vi "Main.vi"(11 "Module Admin":refnum<class "Delacor_lib_QMH_Module Admin.lvclass">) -> ()   [LabVIEW 2020, in "UI User.lvlib"]
doc: "This template is based off of the Queued Message Handler design pattern and the Queued Message Handler project template that ships with LabVIEW.\n\nThe main difference is that the queue is private to this module and communication between modules is performed via Broadcast and Request events.\n\nRequest events are wrapped in public API methods and are handled in the Event Handling Loop (EHL) of this VI. Any module can register for Broadcast events sent by this module. The EHL generates messages based on user interface actions.\n\nThe Message Handling Loop (MHL) processes messages generated by the EHL, or by other messages. The messages are string values, so new messages can be added easily to the Message Cases case structure in the MHL. Each message cluster can also provide an optional value for Message Data, which is a variant that can be converted to whatever message-specific data is required.\n_____\nBased on DQMH Project Template 6.0.0.91."
uses:
  UI User.lvlib
  <vilib>/Delacor/Delacor QMH/Libraries/Module Admin_class/Delacor_lib_QMH_Module Admin.lvclass
  Module Data--cluster.ctl
  Stop Argument--cluster.ctl
  <vilib>/Delacor/Delacor QMH/Libraries/Message Queue_class/Delacor_lib_QMH_Message Queue.lvclass/Delacor_lib_QMH_Message Queue.ctl
  <vilib>/Delacor/Delacor QMH/Libraries/Module Admin_class/Delacor_lib_QMH_Module Admin.lvclass/Delacor_lib_QMH_Module Admin.ctl
  <vilib>/Delacor/Delacor QMH/Libraries/Message Queue_class/Delacor_lib_QMH_Enqueue Message (Single).vi
  <vilib>/Delacor/Delacor QMH/Libraries/Module Admin_class/Delacor_lib_QMH_Get External Launch.vi
  <vilib>/Utility/error.llb/Error Cluster From Error Code.vi
  <vilib>/ErrorRing/Error Ring.xnode
  <vilib>/Delacor/Delacor QMH/Libraries/Message Queue_class/Delacor_lib_QMH_Message Queue.lvclass
  Hardware DAQ/Hardware DAQ.lvlib
  Client HTTP Post/Client HTTP Post.lvlib
  Client HTTP Get/Client HTTP Get.lvlib
panel:
  in  "Radio Buttons Main":T1(radio)
  out "Tab Main":T2(tab)
  out "Active Modules (GET)":string[](array[string])
  in  "ID GET":i32(ring) items=["All"=-1, "1"=1, "2"=2, "3"=3, "4"=4]
  in  "Arrancar - GET":bool
  out "Active Modules (POST)":string[](array[string])
  in  "ID POST":i32(ring) items=["All"=-1, "1"=1, "2"=2, "3"=3]
  in  "Arrancar - POST":bool
  in  "Open Panel DAQ":bool
  in  "Show Panel DAQ":bool
  out "Contador Productos":u16(knob) caption="Gauge" scale=0.0..250.0
  out "DO-3":bool
  out "DO-2":bool
  out "DO-1":bool
  out "DO-0":bool
  in  "Digital Output 3":bool
  in  "Digital Output 2":bool
  in  "Digital Output 1":bool
  in  "Digital Output 0":bool
  out "Digital Inputs":bool[](array[boolean])
  out "Voltimetro - 4":dbl format="%.3f"
  out "Voltimetro - 3":dbl format="%.3f"
  out "Voltimetro - 2":dbl format="%.3f"
  out "Voltimetro - 1":dbl format="%.3f"
  out "Radio Indicador":T3(radio)
  # "Sistema Para Pruebas de Medida (Hardware Embebido,\nHardware Industrial)"
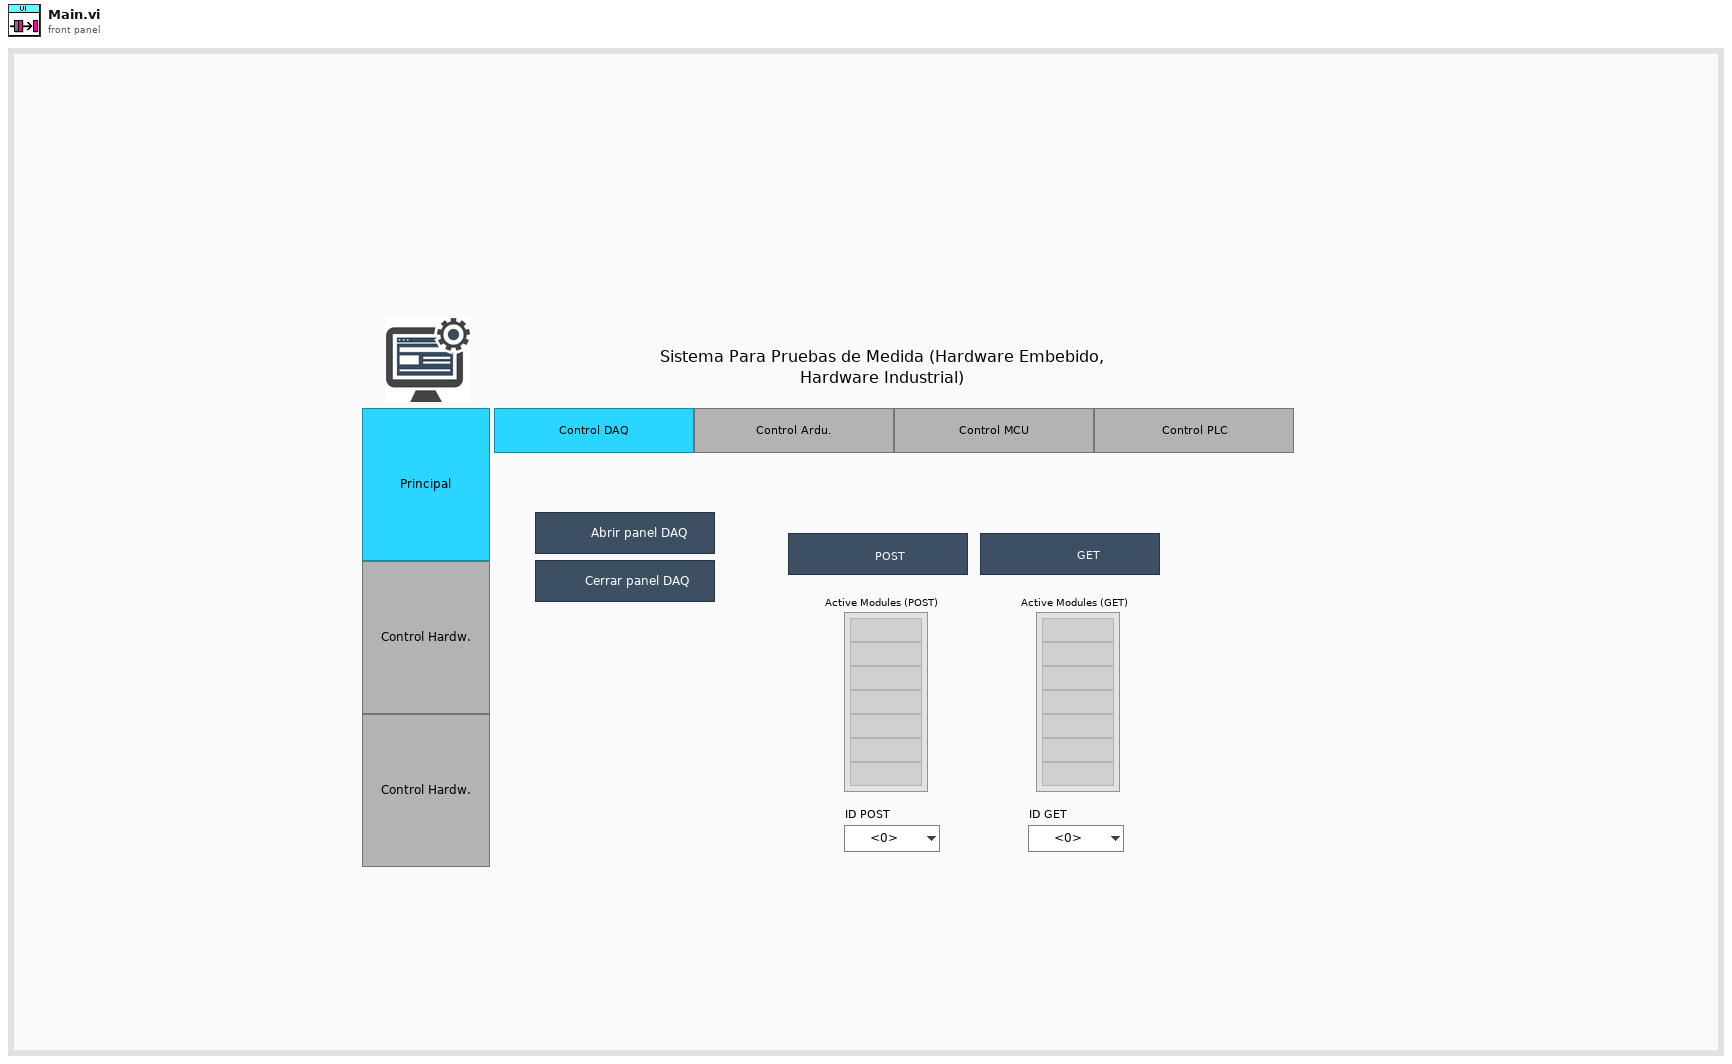
[diagram p1: front panel]
types:
  T1 = enum32{"Principal", "Control Hardware", "Adquisicipon Hardware"}
  T2 = enum32{"Principal", "Control Hardware", "Adquisición Hardware"}
  T3 = enum32{"Control DAQ", "Control Arduino", "Control MCU", "Control PLC"}
  T4 = typedef "UI User.lvlib/Request Events--cluster.ctl" = cluster{"Stop Module":refnum<user-event>, "Show Panel":refnum<user-event>, "Hide Panel":refnum<user-event>, "Get Module Execution Status":refnum<user-event>, "Show Diagram":refnum<user-event>}
  T5 = typedef "UI User.lvlib/Broadcast Events--cluster.ctl" = cluster{"Module Did Init":refnum<user-event>, "Status Updated":refnum<user-event>, "Error Reported":refnum<user-event>, "Module Did Stop":refnum<user-event>, "Update Module Execution Status":refnum<user-event>}
  T6 = typedef "Hardware DAQ.lvlib/Broadcast Events--cluster.ctl" = cluster{"Module Did Init":refnum<user-event>, "Status Updated":refnum<user-event>, "Error Reported":refnum<user-event>, "Module Did Stop":refnum<user-event>, "Update Module Execution Status":refnum<user-event>, "Hardware Connected":refnum<user-event>, "Data Process Volt":refnum<user-event>, "Coil values":refnum<user-event>}
  T7 = typedef "Client HTTP Post.lvlib/Broadcast Events--cluster.ctl" = cluster{"Module Did Init":refnum<user-event>, "Status Updated":refnum<user-event>, "Error Reported":refnum<user-event>, "Did Something":refnum<user-event>, "Module Did Stop":refnum<user-event>, "Update Module Execution Status":refnum<user-event>}
  T8 = typedef "Client HTTP Get.lvlib/Broadcast Events--cluster.ctl" = cluster{"Module Did Init":refnum<user-event>, "Status Updated":refnum<user-event>, "Error Reported":refnum<user-event>, "Did Something":refnum<user-event>, "Module Did Stop":refnum<user-event>, "Update Module Execution Status":refnum<user-event>}
  T9 = cluster{"ID POST":refnum<vi>, "ID GET":refnum<vi>}
  T10 = typedef "UI User.lvlib/Module Data--cluster.ctl" = cluster{"Status":string}
  T11 = enum32{"invalid lock state", "Not Locked", "Locked (No Password)", "Password-protected"}
  T12 = typedef "UI User.lvlib/Stop Argument--cluster.ctl" = cluster{"Origin":string, "Exit via Stop Module Req?":bool, "Wait for Module to stop?":bool}
  T13 = enum32{"Invalid", "Standard", "Closed", "Hidden", "Minimized", "Maximized"}
  T14 = enum16{"DAQ9219", "Arduino", "Xpress Board", "PLC Logo", "Default"}
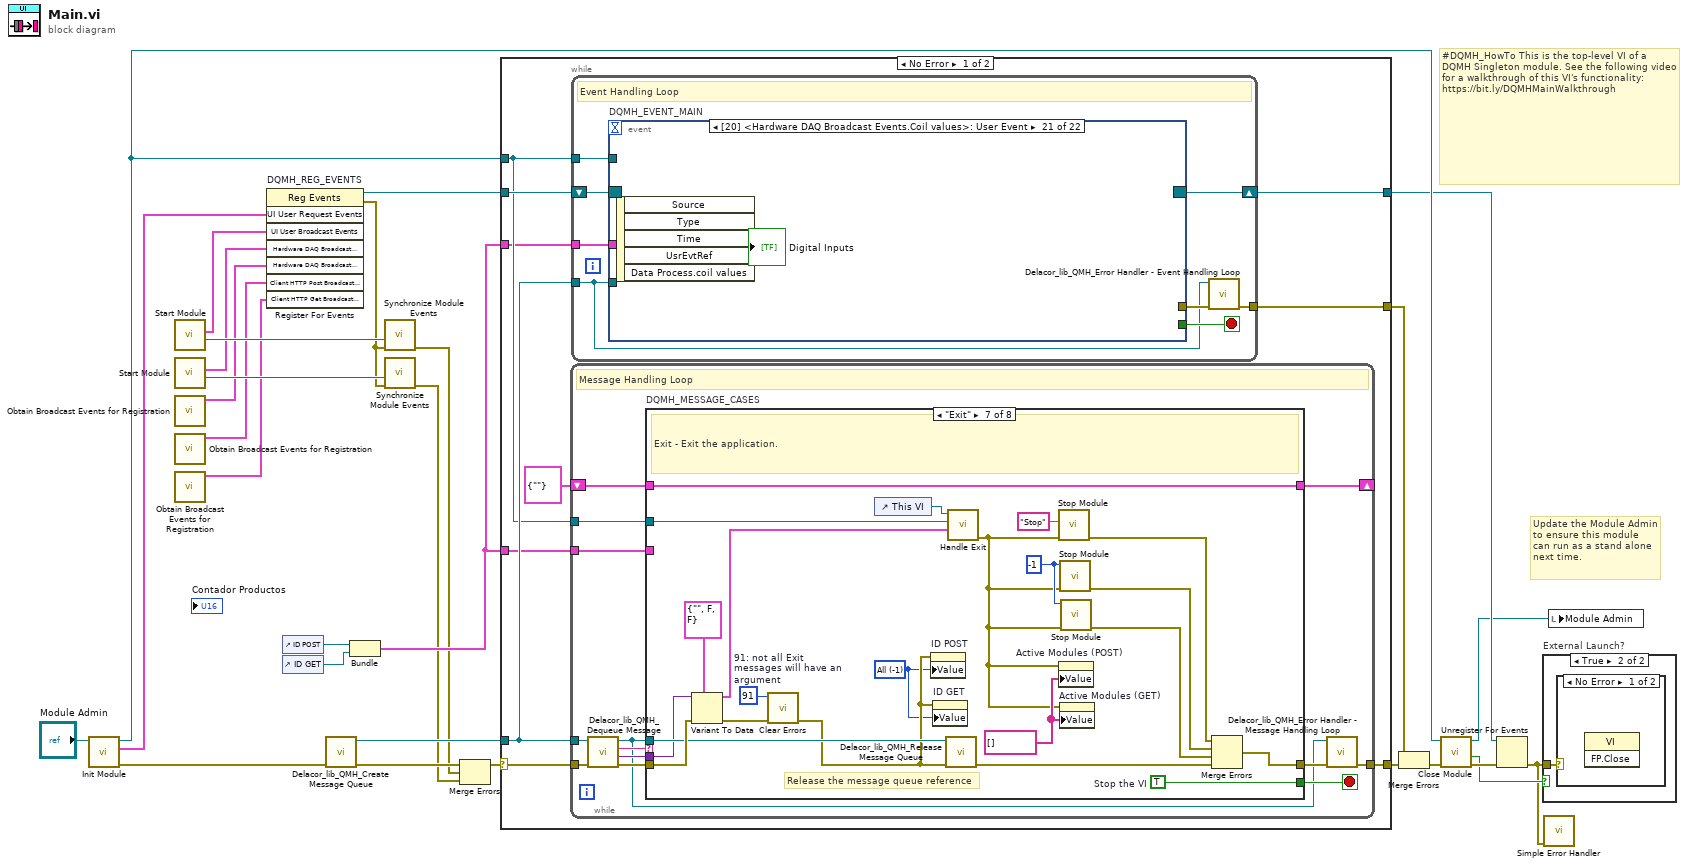
[diagram p0: block diagram]
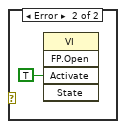
[diagram p3: hidden frame]
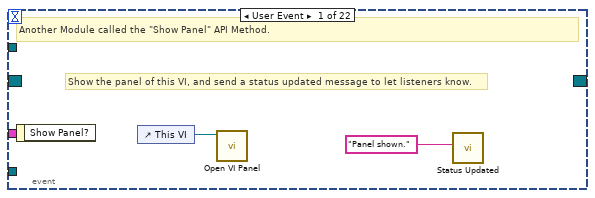
[diagram p4: hidden frame]
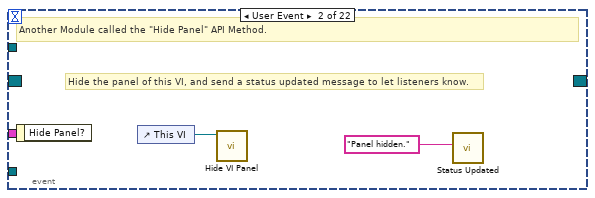
[diagram p5: hidden frame]
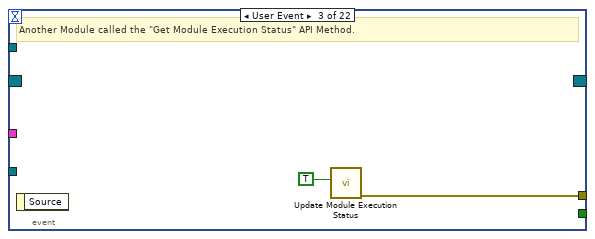
[diagram p6: hidden frame]
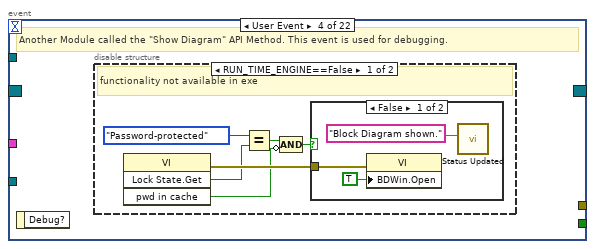
[diagram p7: hidden frame]
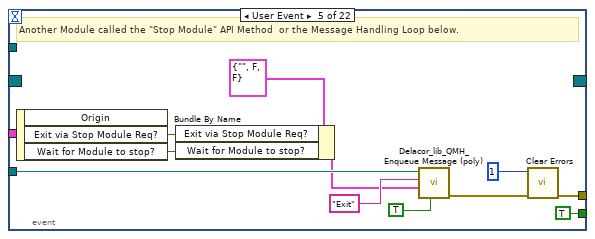
[diagram p10: hidden frame]
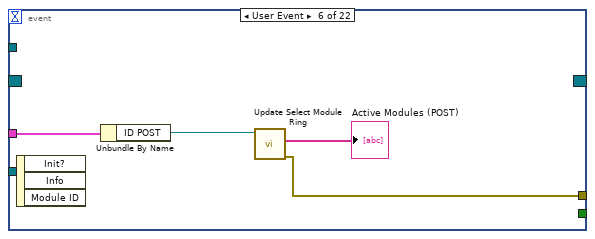
[diagram p11: hidden frame]
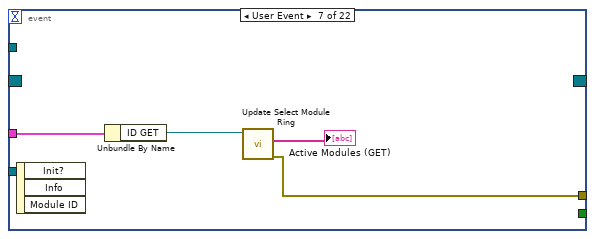
[diagram p12: hidden frame]
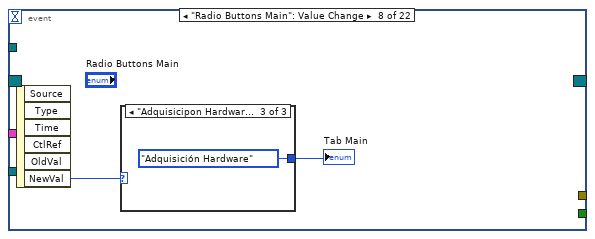
[diagram p13: hidden frame]
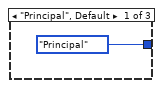
[diagram p14: hidden frame]
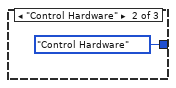
[diagram p15: hidden frame]
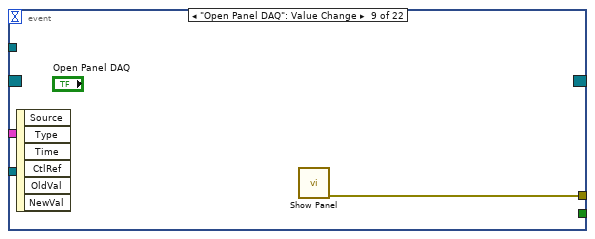
[diagram p16: hidden frame]
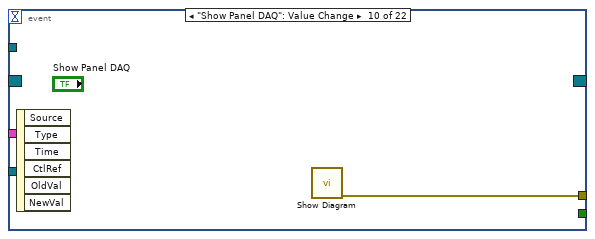
[diagram p17: hidden frame]
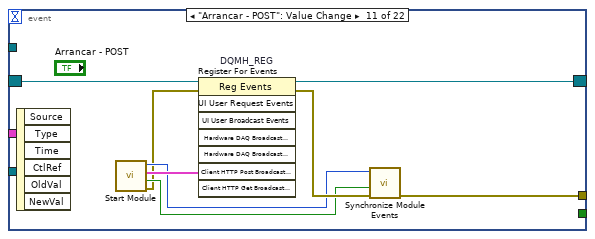
[diagram p18: hidden frame]
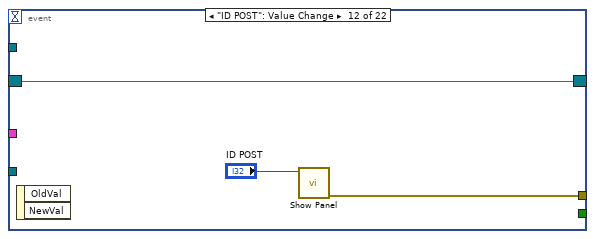
[diagram p19: hidden frame]
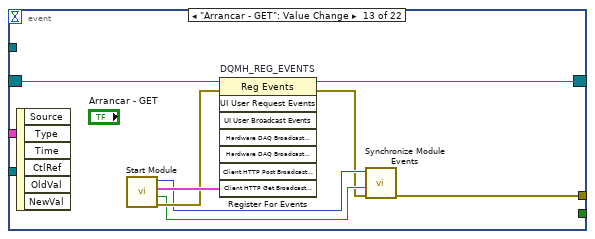
[diagram p20: hidden frame]
diagram:
  # "#DQMH_HowTo This is the top-level VI of a DQMH Singleton module. See the following video for a walkthrough of this VI's functionality: https://bit.ly/DQMHMainWalkthrough"
  # "Update the Module Admin to ensure this module can run as a stand alone next time."
  n1 = call "Init Module.vi"("Singleton Module Admin in"="Module Admin") -> ("error out"=w28:errorcluster, "UI User Request Events"=w19:T4, "Singleton Module Admin out"=w22:refnum<class "Delacor_lib_QMH_Module Admin.lvclass">)  [unwired: 8 in]
  n2 = call "Start Module.vi"() -> ("Wait for Event Sync?"=w8:bool, "UI User Broadcast Events"=w9:T5)  [unwired: 8 in, 2 out]
  n3 = call "Start Module.vi"() -> ("Wait for Event Sync?"=w13:bool, "Hardware DAQ Broadcast Events"=w4:T6)  [unwired: 8 in, 2 out]
  n4 = call "Obtain Broadcast Events for Registration.vi"() -> ("Hardware DAQ Broadcast Events"=w3:T6)  [unwired: 9 in, 2 out]
  n5 = call "Obtain Broadcast Events for Registration.vi"() -> ("Client HTTP Post Broadcast Events"=w2:T7)  [unwired: 9 in, 2 out]
  n6 = call "Obtain Broadcast Events for Registration.vi"() -> ("Client HTTP Get Broadcast Events"=w1:T8)  [unwired: 9 in, 2 out]
  n7 = register-events "DQMH_REG_EVENTS"(w19, w9, w4, w3, w2, w1) -> (reference out=w20:refnum<event-registration>, error out=w7:errorcluster)  [unwired: 2 in]
  n8 = control-ref of="ID POST"() -> (w12:refnum<vi>)
  n9 = control-ref of="ID GET"() -> (w10:refnum<vi>)
  n10 = call <vilib>:"Delacor_lib_QMH_Create Message Queue.vi"("error in"=w28) -> ("error out"=w24:errorcluster, "Message Queue"=w18:refnum<class "Delacor_lib_QMH_Message Queue.lvclass">)  [unwired: 9 in]
  n11 = Bundle("ID POST"=w12, "ID GET"=w10) -> (w11:T9)  [unwired: 1 in]
  n12 = call "Synchronize Module Events.vi"("error in"=w7, "Wait for Event Sync?"=w8) -> ("error out"=w6:errorcluster)  [unwired: 9 in]
  n13 = call "Synchronize Module Events.vi"("error in"=w7, "Wait for Event Sync?"=w13) -> ("error out"=w5:errorcluster)  [unwired: 9 in]
  n14 = Merge Errors(w24, w6, w5) -> (w23:errorcluster)
  n15 = case shown="No Error" w23 {
    selector: w23 -> [w37 w250]
    tunnel: [w39 w249] -> w29
    tunnel: [w36 w255] -> w21
    tunnel: w20 -> [w34 w255]
    tunnel: w18 -> [w33 w248]
    tunnel: [w38 _] -> w26
    tunnel: w22 -> [w32 w251]
    tunnel: w11 -> [w31 _]
    tunnel: w11 -> [w30 _]
    frame No Error {
      n16 = while {
        tunnel: w33 -> [w147]
        shift-right: [w151] -> _
        shift-left: T10 {"Status"=""} ("Data Cluster") -> [w152]
        tunnel: w37 -> [w155]
        tunnel: [w153] -> w39
        tunnel: w32 -> [w145]
        tunnel: w31 -> [w144]
        stop <- w150 stop-if-true
        # "Message Handling Loop"
        n17 = call-dynamic "Delacor_lib_QMH_Dequeue Message.vi"("error in"=w155, "Message Queue in"=w147) -> ("error out"=w154:errorcluster, "Message Data"=w148:variant, "Message"=w149:string, "Message Queue out"=w146:refnum<class "Delacor_lib_QMH_Message Queue.lvclass">)  [unwired: 6 in]
        n18 = case "DQMH_MESSAGE_CASES" shown="\"Exit\"" w149 {
          selector: w149 -> [_ _ _ _ _ _ _ w235]
          tunnel: w146 -> [_ _ _ _ _ w199 w229 _]
          tunnel: w154 -> [w175 w178 w181 w183 w188 w205 w233 w237]
          tunnel: [w157 w178 w180 w183 w187 w196 w231 w238] -> w156
          tunnel: w152 -> [w164 w177 w179 w182 w185 w201 w228 w236]
          tunnel: [w164 w177 w179 w182 w185 w201 w228 w236] -> w151
          tunnel: [_ _ _ _ _ _ w227 _] -> w150
          tunnel: w148 -> [_ _ _ _ _ w200 w226 _]
          tunnel: w145 -> [w168 _ _ _ _ w198 w221 _]
          tunnel: w144 -> [w163 _ _ _ _ _ _ _]
          frame "Initialize" {
            w158 = string[] [] ("Active Modules (POST)")
            w160 = -1 items=["All"=-1] ("ID POST")
            # "Initialize - Any operation that needs to be done before the module can receive messages. Synchronize Caller Events.vi will inform Start Module.vi that the module has launched and is ready to receive messages. Module Did Init.vi will broadcast that the module initialized."
            n19 = call "Synchronize Caller Events.vi"("error in (no error)"=w175, "Singleton Module Admin in"=w168) -> ("error out"=w161:errorcluster, "Singleton Module Admin out"=w165:refnum<class "Delacor_lib_QMH_Module Admin.lvclass">)  [unwired: 8 in]
            n20 = Unbundle By Name(w163) -> ("ID POST"=w162:refnum<vi>)
            n21 = property class="Module Admin"(reference=w165) -> ("Accessors:External Launch"=w172:bool)  [unwired: 1 in, 2 out]
            n22 = call "Init Select Module Ring.vi"("error in (no error)"=w161, "Select Module Ring Ref"=w162) -> ("error out"=w159:errorcluster)  [unwired: 7 in, 2 out]
            n23 = Select(t=T13."Hidden" ("State"), s=w172, f=T13."Standard" ("State")) -> (s? t:f=w169:T13)
            n24 = property on="ID POST" class="Ring (strict)"(error in=w159, "Value"=w160) -> ()  [unwired: 1 in, 2 out]
            n25 = property on="ID GET" class="Ring (strict)"(error in=w159, "Value"=w160) -> ()  [unwired: 1 in, 2 out]
            n26 = call "Module Name--constant.vi"() -> ("Module Name"=w174:string)  [unwired: 11 in]
            n27 = property class="VI"("Front Panel.Title"=w174) -> (reference out=w173:refnum<vi>, error out=w176:errorcluster)  [unwired: 2 in]
            n28 = call "Module Name--constant.vi"() -> ("Module Name"=w166:string)  [unwired: 11 in]
            n29 = invoke class="VI" method="FP.Open"(reference=w173, error in=w176, "State"=w169) -> ()  [unwired: 2 in, 5 out]
            n30 = call "Module Did Init.vi"("error in (no error)"=w161, "Initialized?"=TRUE, "Origin"=w166) -> ("error out"=w157:errorcluster)  [unwired: 8 in]
            n31 = property on="Active Modules (POST)" class="Arr (strict)"(error in=w157, "Value"=w158) -> ()  [unwired: 1 in, 2 out]
            n32 = property on="Active Modules (GET)" class="Arr (strict)"(error in=w157, "Value"=w158) -> ()  [unwired: 1 in, 2 out]
          }
          frame "---Module Specific---" {
            # "Separator -- The following cases handle messages specific to this Module."
          }
          frame "---Copy This Frame---" {
            # "Duplicate this frame when creating new messages.  Change this comment in the duplicated frame to describe this message."
            n33 = Merge Errors(w181) -> (w180:errorcluster)
          }
          frame "---Exit and Error Handling---" {
            # "Separator - The following cases handle errors and exit messages."
          }
          frame "Simulate MHL Error" {
            # "#DQMH_HowTo The 'Simulate MHL Error' button  illustrates how the MHL handles errors. This event is instructional in nature and can be removed."
            # "Simulate an error occurring at the MHL"
            n34 = call "Module Name--constant.vi"() -> ("Module Name"=w184:string)  [unwired: 11 in]
            n35 = xnode "Error Ring"("parameter 0"=w184) -> ("error out"=w186:errorcluster)
            n36 = Merge Errors(w188, w186) -> (w187:errorcluster)
          }
          frame "Error" {
            # "Error - Check the error message data and respond accordingly. This message is sent by the \"Error Handler\" VIs at the end of each loop in this application."
            n37 = property class="Module Admin"(reference=w198) -> ("Accessors:External Launch"=w197:bool)  [unwired: 1 in, 2 out]
            n38 = Variant To Data(error in=w205, type=errorcluster {"status"=FALSE, "code"=0, "source"=""} ("error constant"), Variant=w200) -> (data=w206:errorcluster, error out=w203:errorcluster)
            n39 = call "Error Reported.vi"("Error"=w206) -> ()  [unwired: 10 in, 1 out]
            n40 = case shown="False" w197 {
              tunnel: [w211 _] -> w202
              tunnel: w199 -> [w209 _]
              tunnel: w206 -> [w210 _]
              frame False {
                # "If the module is running standalone, then pop up an error dialog and call the \"Exit\" message."
                n41 = call <vilib>:"Simple Error Handler.vi"("error in (no error)"=w210) -> ()  [unwired: 4 in, 5 out]
                n42 = call-poly <vilib>:"Delacor_lib_QMH_Enqueue Message (poly).vi"("Priority Message? (F)"=TRUE, "Message"="Exit", "Message Queue in"=w209) -> ("error out"=w211:errorcluster)  [unwired: 7 in, 1 out]
              }
              frame True {
                # "If the module was launched externally, calling the Error Reported broadcast VI is the only action performed by the \"Error\" message. The module's caller can then process the error appropriately."
              }
            }
            n43 = Merge Errors(w203, w202) -> (w196:errorcluster)
            n44 = call <vilib>:"Simple Error Handler.vi"("error in (no error)"=w196) -> ()  [unwired: 4 in, 5 out]
          }
          frame "Exit" {
            w213 = string[] [] ("Active Modules (POST)")
            w214 = -1 items=["All"=-1] ("ID POST")
            w217 = -1 ("Module ID")
            w225 = 91  # 91: not all Exit messages will have an argument
            w227 = TRUE  # Stop the VI
            # "Release the message queue reference"
            # "Exit - Exit the application."
            n45 = Variant To Data(error in=w233, type=T12 {"Origin"="", "Exit via Stop Module Req?"=FALSE, "Wait for Module to stop?"=FALSE} ("Stop Argument"), Variant=w226) -> (data=w223:T12, error out=w230:errorcluster)
            n46 = call <vilib>:"Clear Errors.vi"("error in (no error)"=w230, "specific error code to clear (0: all)"=w225) -> ("error out"=w215:errorcluster)  [unwired: 4 in, 1 out]
            n47 = control-ref of="This VI"() -> (w222:refnum<vi>)
            n48 = property on="ID POST" class="Ring (strict)"(error in=w215, "Value"=w214) -> ()  [unwired: 1 in, 2 out]
            n49 = property on="ID GET" class="Ring (strict)"(error in=w215, "Value"=w214) -> ()  [unwired: 1 in, 2 out]
            n50 = call-dynamic "Delacor_lib_QMH_Release Message Queue.vi"("error in"=w215, "Message Queue"=w229) -> ("error out"=w232:errorcluster)  [unwired: 9 in]
            n51 = call "Handle Exit.vi"("Stop Argument"=w223, "Admin in"=w221, "VI reference"=w222) -> ("error out"=w212:errorcluster)  [unwired: 7 in, 1 out]
            n52 = call "Stop Module.vi"("error in"=w212, "Origin"="Stop") -> ("error out"=w219:errorcluster)  [unwired: 9 in]
            n53 = property on="Active Modules (POST)" class="Arr (strict)"(error in=w212, "Value"=w213) -> ()  [unwired: 1 in, 2 out]
            n54 = call "Stop Module.vi"("error in (no error)"=w212, "Module ID"=w217) -> ("error out"=w218:errorcluster)  [unwired: 9 in]
            n55 = property on="Active Modules (GET)" class="Arr (strict)"(error in=w212, "Value"=w213) -> ()  [unwired: 1 in, 2 out]
            n56 = call "Stop Module.vi"("error in (no error)"=w212, "Module ID"=w217) -> ("error out"=w216:errorcluster)  [unwired: 9 in]
            n57 = Merge Errors(w219, w218, w216, w232) -> (w231:errorcluster)
          }
          frame Default {
            # "'Default' case only runs if there is a message that isn't defined in any of the other cases.  Output a programming error."
            n58 = call "Module Name--constant.vi"() -> ("Module Name"=w234:string)  [unwired: 11 in]
            n59 = xnode "Error Ring"("parameter 0"=w235, "parameter 1"=w234) -> ("error out"=w239:errorcluster)
            n60 = Merge Errors(w237, w239) -> (w238:errorcluster)
          }
        }
        n61 = call-dynamic "Delacor_lib_QMH_Error Handler - Message Handling Loop.vi"("error in"=w156, "Message Queue in"=w146) -> ("dup error in"=w153:errorcluster)  [unwired: 8 in, 1 out]
      }
      n62 = while {
        tunnel: w33 -> [w41]
        shift-right: [w44] -> w36
        shift-left: w34 -> [w45]
        tunnel: [w46] -> w38
        tunnel: w32 -> [w42]
        tunnel: w30 -> [w40]
        stop <- w43 stop-if-true
        # "Event Handling Loop"
        n63 = event "DQMH_EVENT_MAIN" shown="[20] <Hardware DAQ Broadcast Events.Coil values>: User Event" {
          selector: w45 -> [_ _ _ _ _ _ _ _ _ _ w95 w97 w106 w108 _ _ _ _ _ _ _ _]
          dyn-events: [_ _ _ _ _ _ _ _ _ _ w90 w97 w100 w108 _ _ _ _ _ _ _ _] -> w44
          timeout: _ -> [_ _ _ _ _ _ _ _ _ _ _ _ _ _ _ _ _ _ _ _ _ _]
          tunnel: [_ _ _ _ TRUE ("Discard?") _ _ _ _ _ _ _ _ _ _ _ _ _ _ _ _ _] -> w43
          tunnel: w41 -> [_ _ _ _ w69 _ _ _ _ _ _ _ _ _ _ _ _ _ _ _ _ w136]
          tunnel: [_ _ w53 _ w72 w75 w79 _ w87 w88 w96 w98 w107 w109 w112 w116 w118 w122 _ _ _ w138] -> w47
          tunnel: w42 -> [_ _ _ _ _ _ _ _ _ _ _ _ _ _ _ _ _ _ _ _ _ w135]
          tunnel: w40 -> [_ _ _ _ _ w77 w81 _ _ _ _ _ _ _ _ _ _ _ _ _ _ _]
          event User Event {
            # "Show the panel of this VI, and send a status updated message to let listeners know."
            # "Another Module called the \"Show Panel\" API Method."
            n64 = event-data() -> ()  [unwired: 1 in, 1 out]
            n65 = control-ref of="This VI"() -> (w49:refnum<vi>)
            n66 = call "Open VI Panel.vi"("VI"=w49) -> ()  [unwired: 10 in, 1 out]
            n67 = call "Status Updated.vi"("Status"="Panel shown." ("format string")) -> ()  [unwired: 10 in, 1 out]
          }
          event User Event {
            # "Hide the panel of this VI, and send a status updated message to let listeners know."
            # "Another Module called the \"Hide Panel\" API Method."
            n68 = event-data() -> ()  [unwired: 1 in, 1 out]
            n69 = control-ref of="This VI"() -> (w51:refnum<vi>)
            n70 = call "Hide VI Panel.vi"("VI"=w51) -> ()  [unwired: 10 in, 1 out]
            n71 = call "Status Updated.vi"("Status"="Panel hidden." ("format string")) -> ()  [unwired: 10 in, 1 out]
          }
          event User Event {
            # "Another Module called the \"Get Module Execution Status\" API Method."
            n72 = event-data() -> ()  [unwired: 1 in, 1 out]
            n73 = call "Update Module Execution Status.vi"("Running?"=TRUE) -> ("error out"=w53:errorcluster)  [unwired: 10 in]
          }
          event User Event {
            # "Another Module called the \"Show Diagram\" API Method. This event is used for debugging."
            n74 = event-data() -> ()  [unwired: 1 in, 1 out]
            n75 = disable-structure shown="RUN_TIME_ENGINE==False" {
              frame condition #0 (active) {
                # "functionality not available in exe"
                n76 = invoke class="VI" method="Lock State.Get"() -> (error out=w59:errorcluster, "Get Lock State"=w58:T11, "pwd in cache"=w55:bool)  [unwired: 4 in, 1 out]
                n77 = Equal?(x=T11."Password-protected", y=w58) -> (x = y?=w56:bool)
                n78 = Compound Arithmetic op=AND(w56, invert w55) -> (w54:bool)
                n79 = case shown="False" w54 {
                  tunnel: w59 -> [w62 _]
                  frame False {
                    n80 = property class="VI"(error in=w62, "BDWin.Open"=TRUE ("Block Diagram Window:Open")) -> ()  [unwired: 1 in, 2 out]
                    n81 = call "Status Updated.vi"("Status"="Block Diagram shown." ("format string")) -> ()  [unwired: 10 in, 1 out]
                  }
                  frame True {
                    # "Password-protected VI, and the password is not in the cache. Do not show the diagram."
                  }
                }
              }
              frame condition #1 {
              }
            }
          }
          event User Event {
            # "Another Module called the \"Stop Module\" API Method  or the Message Handling Loop below."
            n82 = event-data() -> ("Exit via Stop Module Req?"=w65:bool, "Wait for Module to stop?"=w64:bool)  [unwired: 1 in, 1 out]
            n83 = Bundle By Name(cluster=T12 {"Origin"="", "Exit via Stop Module Req?"=FALSE, "Wait for Module to stop?"=FALSE} ("Stop Argument"), "Exit via Stop Module Req?"=w65, "Wait for Module to stop?"=w64) -> (w63:T12)
            n84 = call-poly <vilib>:"Delacor_lib_QMH_Enqueue Message (poly).vi"("Priority Message? (F)"=TRUE, "Message Data"=w63, "Message"="Exit", "Message Queue in"=w69) -> ("error out"=w73:errorcluster)  [unwired: 6 in, 1 out]
            n85 = call <vilib>:"Clear Errors.vi"("error in (no error)"=w73, "specific error code to clear (0: all)"=1) -> ("error out"=w72:errorcluster)  [unwired: 4 in, 1 out]
          }
          event User Event {
            n86 = event-data() -> ()  [unwired: 1 in, 3 out]
            n87 = Unbundle By Name(w77) -> ("ID POST"=w76:refnum<vi>)
            n88 = call "Update Select Module Ring.vi"("Select Module Ring Ref"=w76) -> ("error out"=w75:errorcluster, "Active Modules (Array)"=→"Active Modules (POST)":string[])  [unwired: 8 in, 1 out]
          }
          event User Event {
            n89 = event-data() -> ()  [unwired: 1 in, 3 out]
            n90 = Unbundle By Name(w81) -> ("ID GET"=w80:refnum<vi>)
            n91 = call "Update Select Module Ring.vi"("Select Module Ring Ref"=w80) -> ("error out"=w79:errorcluster, "Active Modules (Array)"=→"Active Modules (GET)":string[])  [unwired: 8 in, 1 out]
          }
          event "Radio Buttons Main": Value Change {
            n92 = event-data() -> ("NewVal"=w83:T1)  [unwired: 1 in, 5 out]
            n93 = case shown="\"Adquisicipon Hardware\"" w83 {
              tunnel: [T2."Principal" ("Tab Main") T2."Control Hardware" ("Tab Main") T2."Adquisición Hardware" ("Tab Main")] -> w82
              frame "Principal", Default {
              }
              frame "Control Hardware" {
              }
              frame "Adquisicipon Hardware" {
              }
            }
            "Tab Main" <- w82
          }
          event "Open Panel DAQ": Value Change {
            n94 = event-data() -> ()  [unwired: 1 in, 6 out]
            n95 = call "Show Panel.vi"() -> ("error out"=w87:errorcluster)  [unwired: 11 in]
          }
          event "Show Panel DAQ": Value Change {
            n96 = event-data() -> ()  [unwired: 1 in, 6 out]
            n97 = call "Show Diagram.vi"() -> ("error out"=w88:errorcluster)  [unwired: 11 in]
          }
          event "Arrancar - POST": Value Change {
            n98 = event-data() -> ()  [unwired: 1 in, 6 out]
            n99 = call "Start Module.vi"() -> ("error out"=w89:errorcluster, "Wait for Event Sync?"=w91:bool, "Client HTTP Post Broadcast Events"=w94:T7, "Module ID"=w92:i32)  [unwired: 8 in]
            n100 = register-events "DQMH_REG"(reference=w95, error in=w89, w94) -> (reference out=w90:refnum<event-registration>, error out=w93:errorcluster)  [unwired: 5 in]
            n101 = call "Synchronize Module Events.vi"("error in"=w93, "Wait for Event Sync?"=w91, "Module ID in"=w92) -> ("error out"=w96:errorcluster)  [unwired: 7 in, 1 out]
          }
          event "ID POST": Value Change {
            n102 = event-data() -> ()  [unwired: 1 in, 2 out]
            n103 = call "Show Panel.vi"("Module ID"="ID POST") -> ("error out"=w98:errorcluster)  [unwired: 10 in]
          }
          event "Arrancar - GET": Value Change {
            n104 = event-data() -> ()  [unwired: 1 in, 6 out]
            n105 = call "Start Module.vi"() -> ("error out"=w104:errorcluster, "Wait for Event Sync?"=w102:bool, "Client HTTP Get Broadcast Events"=w105:T8, "Module ID"=w103:i32)  [unwired: 8 in]
            n106 = register-events "DQMH_REG_EVENTS"(reference=w106, error in=w104, w105) -> (reference out=w100:refnum<event-registration>, error out=w101:errorcluster)  [unwired: 5 in]
            n107 = call "Synchronize Module Events.vi"("error in"=w101, "Wait for Event Sync?"=w102, "Module ID in"=w103) -> ("error out"=w107:errorcluster)  [unwired: 7 in, 1 out]
          }
          event "ID GET": Value Change {
            n108 = event-data() -> ()  [unwired: 1 in, 3 out]
            n109 = call "Show Panel.vi"("Module ID"="ID GET") -> ("error out"=w109:errorcluster)  [unwired: 10 in]
          }
          event "Digital Output 0": Value Change {
            n110 = event-data() -> ()  [unwired: 1 in, 3 out]
            n111 = call "Digital Output 0.vi"("Digital Output 0"="Digital Output 0") -> ("error out"=w112:errorcluster, "Digital Output 0_I"=→"DO-0":bool)  [unwired: 8 in, 1 out]
          }
          event "Digital Output 1": Value Change {
            n112 = event-data() -> ()  [unwired: 1 in, 3 out]
            n113 = call "Digital Output 1.vi"("Digital Output 1"="Digital Output 1") -> ("error out"=w116:errorcluster, "Digital Output 1_I"=→"DO-1":bool)  [unwired: 8 in, 1 out]
          }
          event "Digital Output 2": Value Change {
            n114 = event-data() -> ()  [unwired: 1 in, 3 out]
            n115 = call "Digital Output 2.vi"("Digital Output 2"="Digital Output 2") -> ("error out"=w118:errorcluster, "Digital Output 2_I"=→"DO-3":bool)  [unwired: 8 in, 1 out]
          }
          event "Digital Output 3": Value Change {
            n116 = event-data() -> ()  [unwired: 1 in, 3 out]
            n117 = call "Digital Output 3.vi"("Digital Output 3"="Digital Output 3") -> ("error out"=w122:errorcluster, "Digital Output 3_I"=→"DO-2":bool)  [unwired: 8 in, 1 out]
          }
          event User Event {
            n118 = event-data() -> ("Hardware Connected"=w124:T14)  [unwired: 1 in, 4 out]
            n119 = case shown="\"PLC Logo\"" w124 {
              tunnel: [T3."Control DAQ" ("Radio Indicador") T3."Control Arduino" ("Radio Indicador") T3."Control MCU" ("Radio Indicador") T3."Control PLC" ("Radio Indicador")] -> w123
              frame "DAQ9219", Default {
              }
              frame "Arduino" {
              }
              frame "Xpress Board" {
              }
              frame "PLC Logo" {
              }
            }
            "Radio Indicador" <- w123
          }
          event User Event {
            n120 = event-data() -> ("Data Process.Volt"=w133:dbl[])  [unwired: 1 in, 4 out]
            n121 = Index Array(array=w133) -> (element #1=→"Voltimetro - 1":dbl, element #2=→"Voltimetro - 2":dbl, element #3=→"Voltimetro - 3":dbl, element #4=→"Voltimetro - 4":dbl)  [unwired: 4 in]
          }
          event User Event {
            n122 = event-data() -> ()  [unwired: 1 in, 5 out]
          }
          event Panel Close? {
            w137 = TRUE  # Discard the event, the MHL is responsible for closing and stopping this VI.
            # "Hide the panel or send the 'Exit' message if the user clicks the 'X' on the module main VI panel."
            n123 = event-data() -> ()  [unwired: 1 in, 1 out]
            n124 = property class="Module Admin"(reference=w135) -> ("Accessors:External Launch"=w134:bool)  [unwired: 1 in, 2 out]
            n125 = case shown="False" w134 {
              tunnel: w136 -> [_ w142]
              tunnel: [_ w143] -> w138
              frame True {
                # "If externally launched, clicking the 'X' hides the panel, but doesn't close it."
                n126 = control-ref of="This VI"() -> (w139:refnum<vi>)
                n127 = call "Hide VI Panel.vi"("VI"=w139) -> ()  [unwired: 10 in, 1 out]
              }
              frame False {
                # "If run as a stand-alone VI, clicking the panel 'X' stops the VI."
                n128 = call-poly <vilib>:"Delacor_lib_QMH_Enqueue Message (poly).vi"("Priority Message? (F)"=TRUE, "Message"="Exit", "Message Queue in"=w142) -> ("error out"=w143:errorcluster)  [unwired: 7 in, 1 out]
              }
            }
            n129 = event-data("Discard?"=w137) -> ()  [unwired: 1 in, 1 out]
          }
        }
        n130 = call-dynamic "Delacor_lib_QMH_Error Handler - Event Handling Loop.vi"("error in"=w47, "Message Queue in"=w41) -> ("dup error in"=w46:errorcluster)  [unwired: 8 in, 1 out]
      }
    }
    frame Error {
      # "Synchronize Caller Events.vi will inform Start Module.vi that the module has launched and will let the code calling Start Module.vi register for broadcasts and would permit the caller receive the broadcast that an error occurred at launch time."
      n131 = call-dynamic "Delacor_lib_QMH_Release Message Queue.vi"("error in"=w250, "Message Queue"=w248) -> ("error out"=w249:errorcluster)  [unwired: 9 in]
      n132 = call "Synchronize Caller Events.vi"("Singleton Module Admin in"=w251) -> ("error out"=w256:errorcluster)  [unwired: 9 in, 1 out]
      n133 = call "Module Name--constant.vi"() -> ("Module Name"=w254:string)  [unwired: 11 in]
      n134 = Format Into String(format string="An error occurred during initialization. %s is no longer running.", w254) -> (resulting string=w252:string)  [unwired: 2 in, 1 out]
      n135 = Merge Errors(w249, w256) -> (w257:errorcluster)
      n136 = call "Error Reported.vi"("Additional Information"=w252, "Error"=w257) -> ()  [unwired: 9 in, 1 out]
    }
  }
  n137 = Merge Errors(w26, w29) -> (w25:errorcluster)
  n138 = call "Close Module.vi"("error in (no error)"=w25, "Module Admin in"=w22) -> ("error out"=w27:errorcluster, "External Launch"=w15:bool, "Module Admin out"=w16:refnum<class "Delacor_lib_QMH_Module Admin.lvclass">)  [unwired: 7 in]
  n139 = Unregister For Events(event registration refnum=w21, error in=w27) -> (error out=w14:errorcluster)
  n140 = case "External Launch?" shown="True" w15 {
    tunnel: w14 -> [_ w258]
    frame False {
    }
    frame True {
      n141 = case shown="No Error" w258 {
        frame No Error {
          n142 = invoke class="VI" method="FP.Close"() -> ()  [unwired: 3 in, 3 out]
        }
        frame Error {
          n143 = invoke class="VI" method="FP.Open"("Activate"=TRUE ("Activate?")) -> ()  [unwired: 4 in, 5 out]
        }
      }
    }
  }
  n144 = call <vilib>:"Simple Error Handler.vi"("error in (no error)"=w14) -> ()  [unwired: 4 in, 5 out]
  n145 = local write "Module Admin"(w16) -> ()
